vi "Middle Rail.vi"(11 "Full System Configuration":T1 {"Ballast"."Side" max=5 step=1; "Ballast"."Small" max=5 step=1; "Ballast"."Main" max=5 step=1}) -> (2 "cluster":T5)   [LabVIEW 2023]
uses:
  Option Type Defs/Parts List.ctl
  Option Type Defs/Full System Configuration.ctl
  Option Type Defs/Rack.ctl
  Option Type Defs/Middle Rail.ctl
  Option Type Defs/Ballast.ctl
  <userlib>/_OpenG.lib/lvdata/lvdata.llb/openg_variant.lvlib
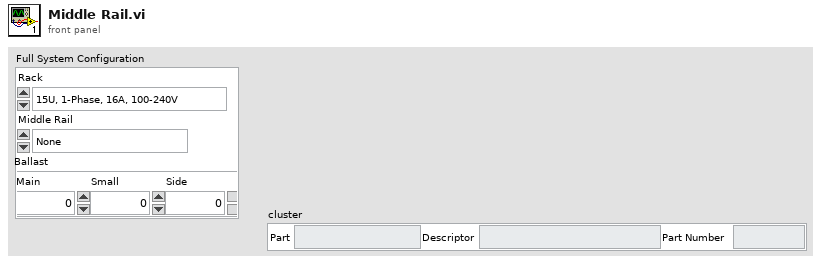
[diagram p1: front panel]
types:
  T1 = typedef "Full System Configuration.ctl" = cluster{"Rack":T2, "Middle Rail":T3, "Ballast":T4}
  T2 = typedef "Rack.ctl" = enum16{"15U, 1-Phase, 16A, 100-240V", "15U, 1-Phase, 24A, 100-240V", "38U, 3-Phase Delta, 50A, 200-240V", "38U, 1-Phase, 24A, 100-120V", "38U, 3-Phase Wye, 50A, 200-240V", "38U, 3-Phase Delta, 50A, 380-480V", "38U, 3-Phase Delta, 32A, 200-240V", "38U, 3-Phase Wye, 16A, 100-240V", "44U, 1-Phase, 24A, 100-240V", "44U, 3-Phase Delta, 32A, 200-240V"}
  T3 = typedef "Middle Rail.ctl" = enum16{"None", "Flip Side Rear, D=168.83mm", "Parallel Rear, D=145mm", "Flip Side Front, D=145mm", "Parallel Front, D=145mm"}
  T4 = typedef "Ballast.ctl" = cluster{"Main":u16, "Small":u16, "Side":u16}
  T5 = typedef "Parts List.ctl" = cluster{"Part":string, "Descriptor":string, "Part Number":string}
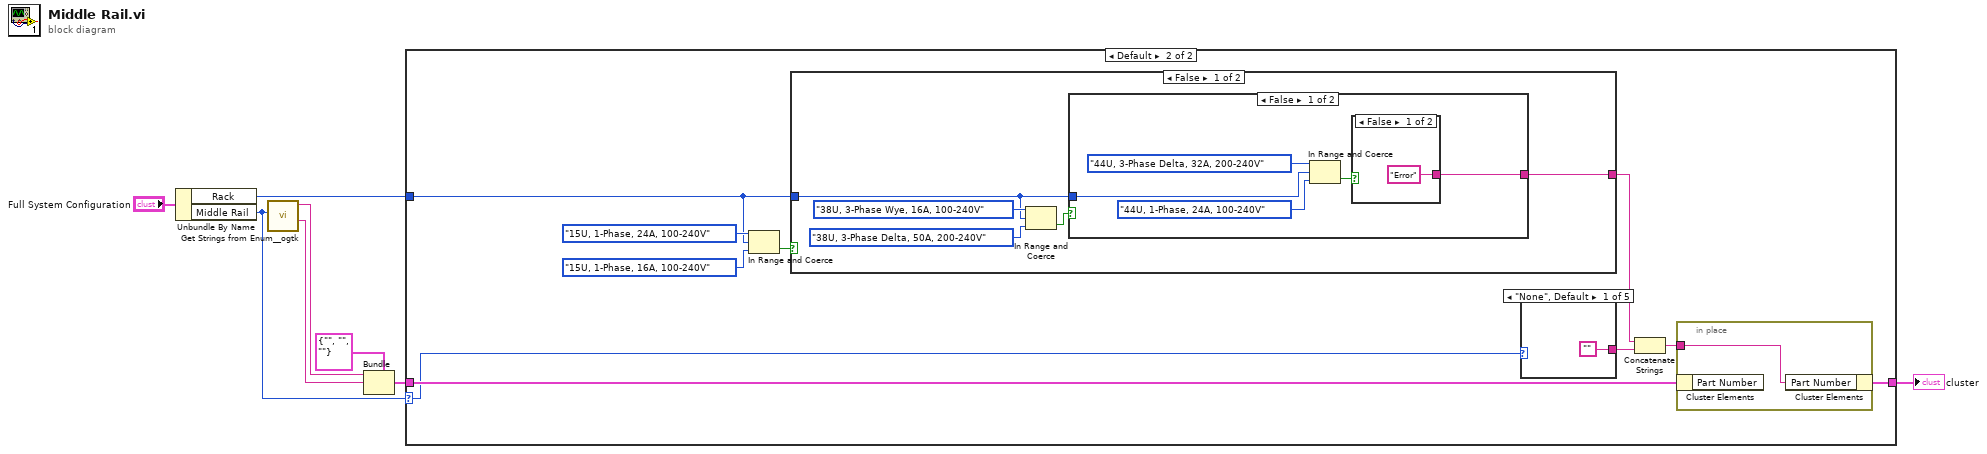
[diagram p0: block diagram]
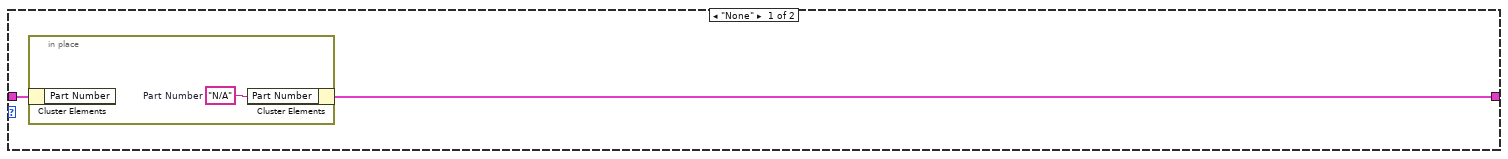
[diagram p2: hidden frame]
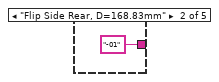
[diagram p3: hidden frame]
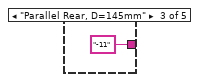
[diagram p4: hidden frame]
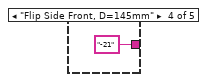
[diagram p5: hidden frame]
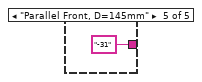
[diagram p6: hidden frame]
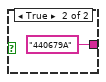
[diagram p7: hidden frame]
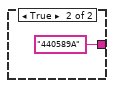
[diagram p8: hidden frame]
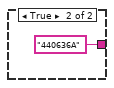
[diagram p9: hidden frame]
diagram:
  n1 = Unbundle By Name("Full System Configuration") -> ("Rack"=w7:T2, "Middle Rail"=w6:T3)
  n2 = call <userlib>:"Get Strings from Enum__ogtk.vi"("Enum"=w6) -> ("String Value"=w4:string, "Enum Name"=w3:string)  [unwired: 7 in, 2 out]
  n3 = Bundle(cluster=T5 {"Part"="", "Descriptor"="", "Part Number"=""}, "Part"=w3, "Descriptor"=w4) -> (w5:T5)  [unwired: 1 in]
  n4 = case shown="Default" w6 {
    selector: w6 -> [_ w16]
    tunnel: w5 -> [w10 w21]
    tunnel: w7 -> [_ w12]
    tunnel: [w9 w18] -> w8
    frame "None" {
      n5 = in-place {
        w11 = "N/A"  # Part Number
        n6 = in-place-cluster #1(w10) -> ()  [unwired: 1 out]
        n7 = in-place-cluster #1("Part Number"=w11) -> (w9:T5)
      }
    }
    frame Default {
      n8 = In Range and Coerce(upper limit=Rack."15U, 1-Phase, 24A, 100-240V" ("Rack"), x=w12, lower limit=Rack."15U, 1-Phase, 16A, 100-240V" ("Rack")) -> (In Range?=w13:bool)  [unwired: 1 out]
      n9 = case shown="False" w13 {
        tunnel: [w31 "440636A"] -> w20
        tunnel: w12 -> [w27 _]
        frame False {
          n10 = In Range and Coerce(upper limit=Rack."38U, 3-Phase Wye, 16A, 100-240V" ("Rack"), x=w27, lower limit=Rack."38U, 3-Phase Delta, 50A, 200-240V" ("Rack")) -> (In Range?=w28:bool)  [unwired: 1 out]
          n11 = case shown="False" w28 {
            tunnel: [w32 "440589A"] -> w31
            tunnel: w27 -> [w34 _]
            frame False {
              n12 = In Range and Coerce(upper limit=Rack."44U, 3-Phase Delta, 32A, 200-240V" ("Rack"), x=w34, lower limit=Rack."44U, 1-Phase, 24A, 100-240V" ("Rack")) -> (In Range?=w33:bool)  [unwired: 1 out]
              n13 = case shown="False" w33 {
                tunnel: ["Error" "440679A"] -> w32
                frame False {
                }
                frame True {
                }
              }
            }
            frame True {
            }
          }
        }
        frame True {
        }
      }
      n14 = case shown="\"None\", Default" w16 {
        tunnel: ["" "-01" "-11" "-21" "-31"] -> w17
        frame "None", Default {
        }
        frame "Flip Side Rear, D=168.83mm" {
        }
        frame "Parallel Rear, D=145mm" {
        }
        frame "Flip Side Front, D=145mm" {
        }
        frame "Parallel Front, D=145mm" {
        }
      }
      n15 = Concatenate Strings(w20, w17) -> (w19:string)
      n16 = in-place {
        in-place-border: w19 -> [w41]
        n17 = in-place-cluster #2(w21) -> ()  [unwired: 1 out]
        n18 = in-place-cluster #2("Part Number"=w41) -> (w18:T5)
      }
    }
  }
  "cluster" <- w8
